vi "GPS.vi"(1 "GPS In":cluster{"X":dbl, "Y":dbl, "Angle ":i16}, 2 "Y":dbl) -> (0 "GPS Out":cluster{"X":dbl, "Y":dbl, "Angle ":i16})   [LabVIEW 2020]
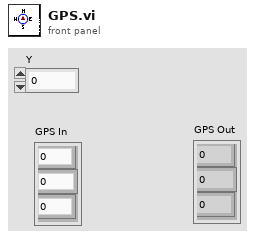
[diagram p1: front panel]
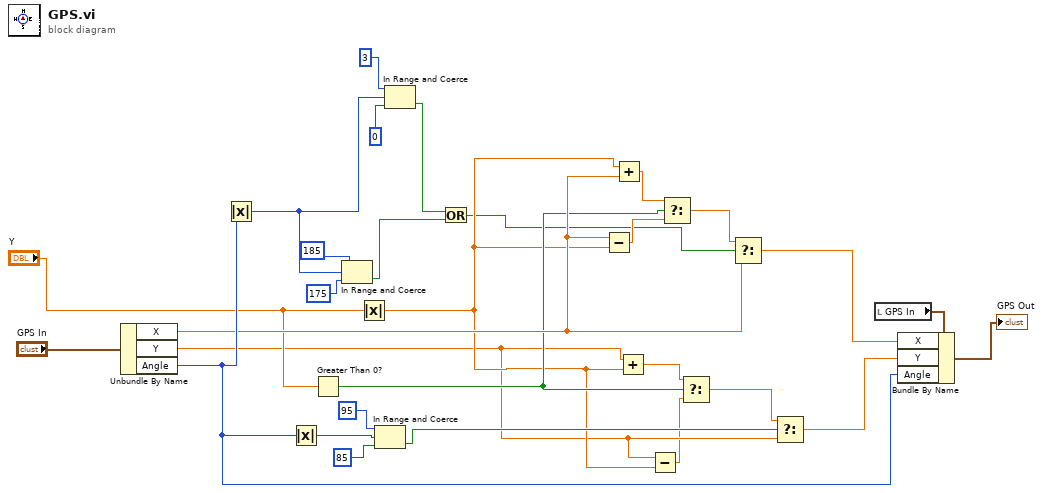
[diagram p0: block diagram]
diagram:
  n1 = Unbundle By Name("GPS In") -> ("X"=w17:dbl, "Y"=w10:dbl, "Angle"=w20:i16)
  n2 = Absolute Value(x=w20) -> (abs(x)=w29:i16)
  n3 = Absolute Value(x=w20) -> (abs(x)=w28:i16)
  n4 = Greater Than 0?(x="Y") -> (x > 0?=w15:bool)
  n5 = In Range and Coerce(upper limit=i16 185, x=w29, lower limit=i16 175) -> (In Range?=w7:bool)  [unwired: 1 out]
  n6 = Absolute Value(x="Y") -> (abs(x)=w11:dbl)
  n7 = In Range and Coerce(upper limit=i16 95, x=w28, lower limit=i16 85) -> (In Range?=w12:bool)  [unwired: 1 out]
  n8 = In Range and Coerce(upper limit=i16 3, x=w29, lower limit=i16 0 ("abs(x)")) -> (In Range?=w8:bool)  [unwired: 1 out]
  n9 = Or(x=w8, y=w7) -> (x .or. y?=w6:bool)
  n10 = Subtract(x=w17, y=w11) -> (x-y=w18:dbl)
  n11 = Add(x=w11, y=w17) -> (x+y=w19:dbl)
  n12 = Add(x=w10, y=w11) -> (x+y=w25:dbl)
  n13 = Subtract(x=w10, y=w11) -> (x-y=w9:dbl)
  n14 = Select(t=w19, s=w15, f=w18) -> (s? t:f=w27:dbl)
  n15 = Select(t=w25, s=w15, f=w9) -> (s? t:f=w26:dbl)
  n16 = Select(t=w27, s=w6, f=w17) -> (s? t:f=w21:dbl)
  n17 = Select(t=w26, s=w12, f=w10) -> (s? t:f=w23:dbl)
  n18 = local read "GPS In"() -> (w22:cluster{"X":dbl, "Y":dbl, "Angle ":i16})
  n19 = Bundle By Name(cluster=w22, "X"=w21, "Y"=w23, "Angle"=w20) -> (→"GPS Out":cluster{"X":dbl, "Y":dbl, "Angle ":i16})
